vi "SPC_enable_sequencer.vi"(6 "Enable":i16 max=2 step=1, 8 "Error In":errorcluster, 10 "Module No":i16 min=0 max=7 step=1, 11 "DLL Path":path) -> (0 "Error Out":errorcluster, 2 "Module No":i16 min=0 max=7 step=1, 3 "DLL Path":path)   [LabVIEW 2017]
doc: "The procedure is used to enable or disable the sequencer of the SPC module 'mod_no'.\nIf 'mod_no' = -1, sequencer will be enabled/disabled for all SPC modules which are actually in use.\nIf enable = 0:\nIf the sequencer is running:\n - The sequencer is stopped and disabled,\n - The SPC is disarmed (photon collection is stopped),\nIf the sequencer was enabled:\n- The sequencer is disabled\n- The dead time compensation of collection timer is switched to the state specified in the \nsystem parameters\nWhen enable = 1 or 2:\nIf the sequencer was not enabled:\n - The sequencer is enabled\n - The dead time compensation of the collection timer is switched off\nThe way of enabling sequencer ( 'enable' = 1 or 2 ) changes slightly the action of \nSPC_start_measurement function for sequencer operation on SPC-130/6x0/150/131. When \n'enable' =1, SPC_start_measurement arms SPC for both memory banks, while for 'enable' = \n2, the function arms SPC only for current memory bank. \nThe 2nd case is used by the main software to program Continuous Flow measurements with \naccumulation.\nThe sequencer must be enabled before starting the measurement in the following cases:\n- Continuous flow measurements for SPC modules 13x/15x/160 and 6x0 - normal \noperation (routing in ) with sequencer \n- scanning modes ( Scan In , Scan Out ) for SPC modules 7x0, 830, 140, 930, 15x, \n160 )\n- Continuous flow in Scan In mode for SPC-15x/160 module\n- block address out mode for SPC modules 7x0 \n\ninfo@becker-hickl.com"
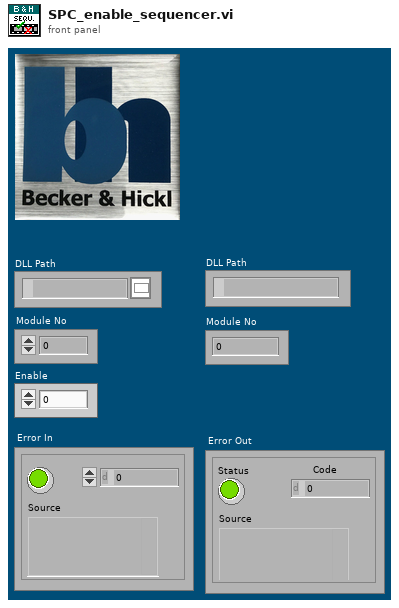
[diagram p1: front panel]
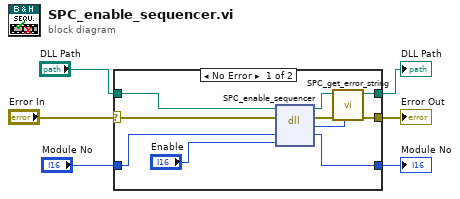
[diagram p0: block diagram]
diagram:
  n1 = case shown="No Error" "Error In" {
    selector: "Error In" -> [w16 w19]
    tunnel: [w12 w19] -> w5
    tunnel: "DLL Path" -> [w15 w18]
    tunnel: [w11 w18] -> w3
    tunnel: "Module No" -> [w9 w17]
    tunnel: [w8 w17] -> w1
    frame No Error {
      n2 = dll-call lib="D:/spcm/lib/lab_view/lv10.0/spcm32.dll" fn="SPC_enable_sequencer"(path in=w15, error in=w16, "mod_no"=w9, "enable"="Enable") -> (path out=w14:path, error out=w13:errorcluster, "return type"=w10:i16, "mod_no"=w8:i16)  [unwired: 2 in]
      n3 = call "SPC_get_error_string.vi"("ErrorID"=w10, "Error In"=w13, "DLL Path"=w14) -> ("Error Out"=w12:errorcluster, "DLL Path"=w11:path)  [unwired: 6 in, 1 out]
    }
    frame Error {
    }
  }
  "Error Out" <- w5
  "DLL Path" <- w3
  "Module No" <- w1
